vi "Add Terminal Status Channel.vi"(8 "error in":errorcluster, 11 "terminal":T1 format="%.0x") -> (0 "error out":errorcluster, 2 "status channel":T1 format="%.0x", 3 "terminal out":T1 format="%.0x")   [LabVIEW 2020, in "AIM MIL-STD-1553 Scripting.lvlib"]
doc: "Adds a <b>status channel</b> to the specified <b>terminal</b>."
uses:
  AIM MIL-STD-1553 Scripting.lvlib
  <vilib>/NI VeriStand/Custom Device API/Custom Device Item Ref.ctl
  <vilib>/NI VeriStand/Custom Device API/Custom Device Channel.ctl
  <vilib>/NI VeriStand/Custom Device API/Custom Device Channel Type.ctl
  Constants.vi
  <vilib>/NI VeriStand/Custom Device API/Custom Device API.lvlib
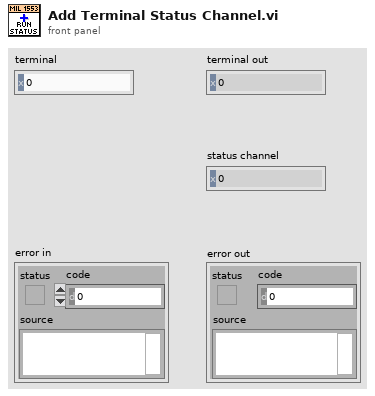
[diagram p1: front panel]
types:
  T1 = typedef "Custom Device API.lvlib/Custom Device Item Ref.ctl" = u64
  T2 = typedef "Custom Device API.lvlib/Custom Device Channel.ctl" = cluster{"Type":T3, "Units":string, "Default Value":dbl, "Faultable":bool, "Scalable":bool}
  T3 = typedef "Custom Device API.lvlib/Custom Device Channel Type.ctl" = enum16{"Input", "Output"}
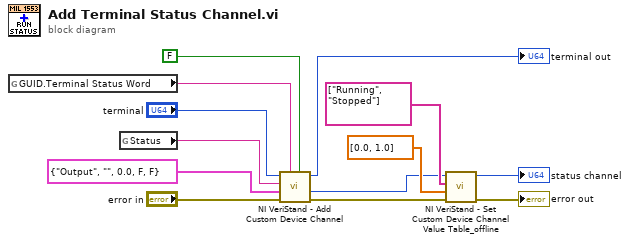
[diagram p0: block diagram]
diagram:
  n1 = global read "Constants.vi" "GUID.Terminal Status Word"() -> (w9:string)
  n2 = global read "Constants.vi" "Status"() -> (w8:string)
  n3 = call <vilib>:"NI VeriStand - Add Custom Device Channel.vi"("Highlight? (F)"=FALSE, "GUID (Default Channel)"=w9, "error in (no error)"="error in", "Channel"=T2 {"Type"=enum."Output", "Units"="", "Default Value"=0.0, "Faultable"=FALSE, "Scalable"=FALSE}, "Channel Name"=w8, "Parent Ref in"="terminal") -> ("error out"=w7:errorcluster, "Channel Ref"=w1:T1, "Parent Ref out"=→"terminal out":T1)  [unwired: 2 in, 1 out]
  n4 = call "NI VeriStand - Set Custom Device Channel Value Table_offline.vi"("error in (no error)"=w7, "Values"=dbl[] [0.0, 1.0] ("RT values"), "Names"=string[] ["Running", "Stopped"] ("RT names"), "Channel Ref in"=w1) -> ("error out"=→"error out":errorcluster, "Channel Ref out"=→"status channel":T1)  [unwired: 6 in]
